vi "CryoServer Make Table From Map.vi"(10 "Ch Map":map{string, T1}(c390), 11 "Telem":T2) -> (3 "table":string[][](array[string]))   [LabVIEW 2024, in "CryoServer.lvclass"]
uses:
  CryoServer.lvclass
  CryoServer Telemetry Map.ctl
  CryoServer Channel Mapping.ctl
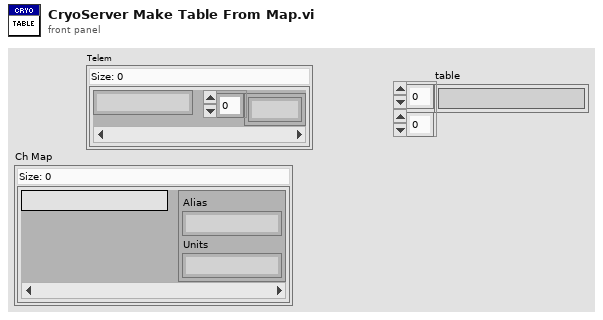
[diagram p1: front panel]
types:
  T1 = typedef "CryoServer Channel Mapping.ctl" = cluster{"Alias":string, "Units":string}
  T2 = typedef "CryoServer Telemetry Map.ctl" = map{string, dbl[]}
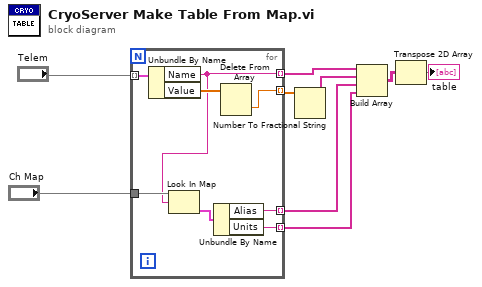
[diagram p0: block diagram]
diagram:
  n1 = for {
    tunnel: "Telem" -> [w17] mode=indexing
    tunnel: [w13] -> w8 mode=indexing
    tunnel: [w15] -> w9 mode=indexing
    tunnel: "Ch Map" -> [w14]
    tunnel: [w11] -> w2 mode=indexing
    tunnel: [w10] -> w1 mode=indexing
    n2 = Unbundle By Name(w17) -> ("Name"=w13:string, "Value"=w16:dbl[])
    n3 = Look In Map(map=w14, key=w13) -> (value=w12:T1)  [unwired: 1 in, 1 out]
    n4 = Unbundle By Name(w12) -> ("Alias"=w11:string, "Units"=w10:string)
    n5 = Delete From Array(array=w16) -> (deleted portion=w15:dbl)  [unwired: 2 in, 1 out]
  }
  n6 = Number To Fractional String(number=w9) -> (F-format string=w7:string[])  [unwired: 3 in]
  n7 = Build Array(w8, w7, w2, w1) -> (w6:string[][])
  n8 = Transpose 2D Array(2D array=w6) -> (transposed array=→"table":string[][])
